vi "start.vi"(8 "error in (no error)":errorcluster, 11 "TrajectoryMG100122GenericFPGA in":refnum<class "TrajectoryMG100122GenericFPGA.lvclass">) -> (0 "error out":errorcluster, 3 "TrajectoryMG100122GenericFPGA out":refnum<class "TrajectoryMG100122GenericFPGA.lvclass">)   [LabVIEW 2010, in "TrajectoryMG100122GenericFPGA.lvclass"]
uses:
  TrajectoryMG100122GenericFPGA.lvclass
  FPGAWrapper/GenericFPGAWrapper/GenericFPGAWrapper/GenericFPGAWrapper.lvclass
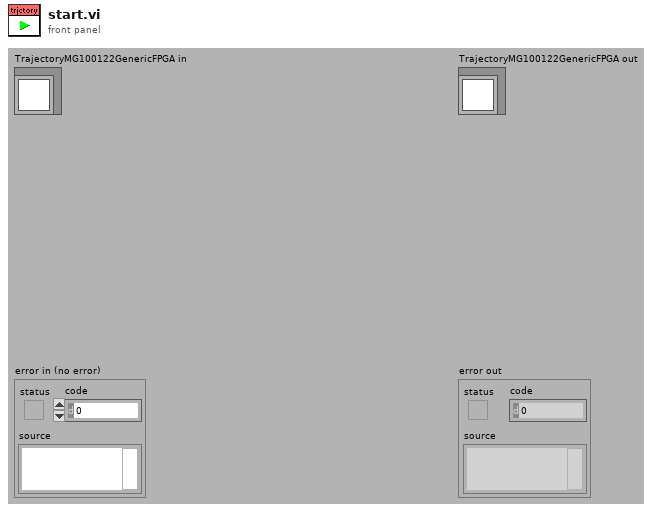
[diagram p1: front panel]
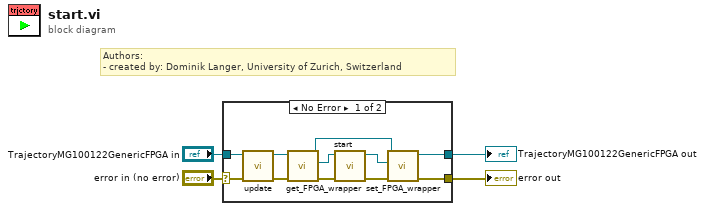
[diagram p0: block diagram]
diagram:
  # "Authors: \n- created by: Dominik Langer, University of Zurich, Switzerland"
  n1 = case shown="No Error" "error in (no error)" {
    selector: "error in (no error)" -> [w6 w17]
    tunnel: [w14 w17] -> w3
    tunnel: [w12 w16] -> w1
    tunnel: "TrajectoryMG100122GenericFPGA in" -> [w8 w16]
    frame No Error {
      n2 = call-dynamic "update.vi"("error in (no error)"=w6, "TrajectoryMG100122GenericFPGA in"=w8) -> ("error out"=w5:errorcluster, "TrajectoryMG100122GenericFPGA out"=w7:refnum<class "TrajectoryMG100122GenericFPGA.lvclass">)  [unwired: 8 in]
      n3 = call-dynamic "get_FPGA_wrapper.vi"("error in (no error)"=w5, "TrajectoryMG100122GenericFPGA in"=w7) -> ("error out"=w10:errorcluster, "GenericFPGAWrapper.lvclass"=w9:refnum<class "GenericFPGAWrapper.lvclass">, "TrajectoryMG100122GenericFPGA out"=w11:refnum<class "TrajectoryMG100122GenericFPGA.lvclass">)  [unwired: 7 in]
      n4 = call-dynamic "start.vi"("error in (no error)"=w10, "GenericFPGAWrapper in"=w9) -> ("error out"=w15:errorcluster, "GenericFPGAWrapper out"=w13:refnum<class "GenericFPGAWrapper.lvclass">)  [unwired: 8 in]
      n5 = call-dynamic "set_FPGA_wrapper.vi"("error in (no error)"=w15, "GenericFPGAWrapper.lvclass"=w13, "TrajectoryMG100122GenericFPGA in"=w11) -> ("error out"=w14:errorcluster, "TrajectoryMG100122GenericFPGA out"=w12:refnum<class "TrajectoryMG100122GenericFPGA.lvclass">)  [unwired: 7 in]
    }
    frame Error {
    }
  }
  "error out" <- w3
  "TrajectoryMG100122GenericFPGA out" <- w1
